vi "FUG-HCN.SetVoltage.vi"(0 "i ref in":refnum<vi>, 2 "Set Voltage":dbl format="%.5f", 4 "Time out":i32, 5 "error in (no error)":errorcluster) -> (14 "i ref out":refnum<vi>, 16 "timed out":bool, 19 "error out":errorcluster)   [LabVIEW 2014, in "FUG-HCN.lvlib"]
doc: "Sets the Voltage at the Device. but first one should increase the current to set the voltage else the Voltage might not be set"
uses:
  FUG-HCN.lvlib
  CS_Core/CSSystem/CoreLib/CoreLib.lvlib
  CS_Core/CSSystem/CoreDefs/CoreDefs.error_type.ctl
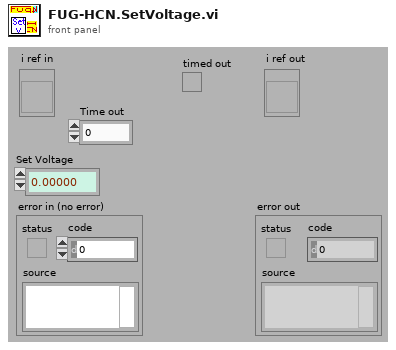
[diagram p1: front panel]
types:
  T1 = typedef "CoreDefs.error_type.ctl" = enum16{"no error", "can't load process", "can't unload process", "process does not exist", "can't install process", "can't remove process", "unknown function", "time out", "can't execute function", "duplicate queue name", "super not found", "caller queue invalid", "can't ping process", "unknown error", "VISA Error", "VISA timeout", "GPIB timeout", "GPIB error", "communication error", "data type mismatch", "can't read data from OPC server", "can't write data to OPC server", "OET error", "function not implemented", "process already exists", "invalid Shared Variable name", "error writing Shared Variable", "error reading Shared Variable", "invalid client name", "corrupt database", "unknown class", "call not authorized", "parameter out of range", "OET timeout: can't get data to modify", "invalid queue name", "requested operation incompatible with current state", "event undefined", "event disabled", "state undefined", "caller is not a friend", "EventBuilder: bad eventID", "EventBuilder: no DAQ devices", "a thread must not stop itself", "UNUSED ELEMENT4", "DiscArchiver: eventData incomplete", "DiscArchiver: eventData does not belong to run", "DiscArchiver: can't open file", "DiscArchiver: can't write to file", "DiscArchiver: available disc space low", "can't acquire semaphore", "error reading data from database", "notifier object is not existing", "can't register process", "can't unregister process", "illegal event type", "object disabled", "object already exists", "can't change state", "Instrument not found", "no connection to remote node", "invalid reference", "N/A", "UNUSED ELEMENT 1", "element not found", "illegal TCP/IP connection detected", "object does not exist", "invalid access ID", "unknown CS system", "invalid privilige", "unsupported data type", "unsupported server type", "IO server already exists", "Shared Variable already exists"}
  T2 = typedef "FUG-HCN.lvlib/FUG-HCN.i attribute.ctl" = cluster{"SetStatus":bool, "Set Voltage":dbl, "Nom Voltage":dbl, "VoltageID":i32, "CurrentID":i32}
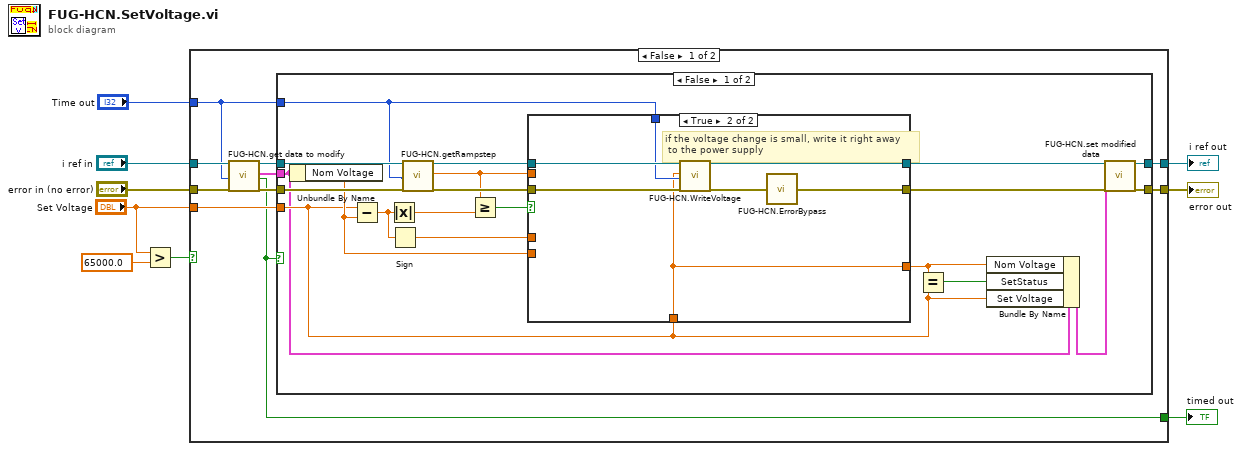
[diagram p0: block diagram]
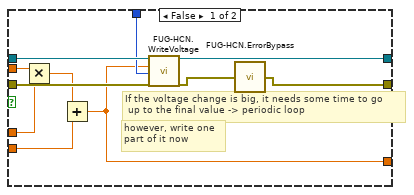
[diagram p2: hidden frame]
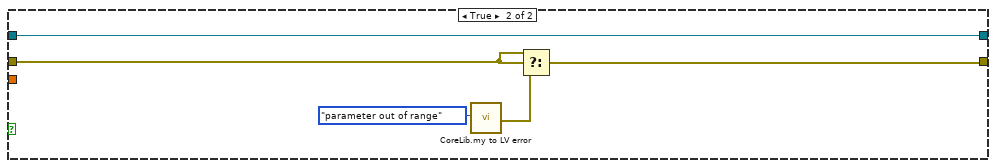
[diagram p4: hidden frame]
diagram:
  n1 = Greater?(x="Set Voltage", y=65000.0) -> (0:w2:bool)
  n2 = case shown="False" w2 {
    tunnel: [w19 w60] -> w9
    tunnel: "Set Voltage" -> [w18 _]
    tunnel: [w17 w64] -> w6
    tunnel: "i ref in" -> [w15 w64]
    tunnel: "error in (no error)" -> [w13 w62]
    tunnel: "Time out" -> [w14 _]
    tunnel: [w10 _] -> w1
    frame False {
      n3 = call "FUG-HCN.get data to modify.vi"("i ref in"=w15, "ms timeout (10000)"=w14, "error in (no error)"=w13) -> ("i ref out"=w16:refnum<vi>, "i attribute"=w11:T2, "timed out"=w10:bool, "error out"=w12:errorcluster)  [unwired: 13 in]
      n4 = case shown="False" w10 {
        tunnel: w11 -> [w22 _]
        tunnel: w12 -> [w33 w58]
        tunnel: [w35 w58] -> w19
        tunnel: w18 -> [w23 _]
        tunnel: w16 -> [w34 w59]
        tunnel: [w39 w59] -> w17
        tunnel: w14 -> [w24 _]
        frame False {
          n5 = Unbundle By Name(w22) -> ("Nom Voltage"=w25:dbl)
          n6 = Subtract(x=w23, y=w25) -> (x-y=w27:dbl)
          n7 = Absolute Value(x=w27) -> (abs(x)=w32:dbl)
          n8 = Sign(1:w27) -> (0:w26:dbl)
          n9 = call "FUG-HCN.getRampstep.vi"("i ref in"=w34, "ms timeout (100)"=w24, "error in (no error)"=w33) -> ("i ref out"=w29:refnum<vi>, "Ramp Step(V)"=w28:dbl, "error out"=w30:errorcluster)  [unwired: 13 in, 1 out]
          n10 = Greater Or Equal?(x=w28, y=w32) -> (x >= y?=w31:bool)
          n11 = case shown="True" w31 {
            tunnel: [w43 w54] -> w38
            tunnel: [w40 w51] -> w37
            tunnel: w30 -> [w49 w55]
            tunnel: w29 -> [w50 w57]
            tunnel: w24 -> [w48 w56]
            tunnel: w23 -> [_ w53]
            tunnel: w28 -> [w47 _]
            tunnel: w26 -> [w46 _]
            tunnel: w25 -> [w44 _]
            tunnel: [w42 w53] -> w21
            frame False {
              # "however, write one\npart of it now"
              # "If the voltage change is big, it needs some time to go\n up to the final value -> periodic loop"
              n12 = Multiply(x=w47, y=w46) -> (x*y=w45:dbl)
              n13 = Add(x=w45, y=w44) -> (x+y=w42:dbl)
              n14 = call "FUG-HCN.WriteVoltage.vi"("i ref in"=w50, "Set Voltage"=w42, "ms timeout (100)"=w48, "error in (no error)"=w49) -> ("i ref out"=w43:refnum<vi>, "error out"=w41:errorcluster)  [unwired: 13 in, 1 out]
              n15 = call "FUG-HCN.ErrorBypass.vi"("error in (no error)"=w41) -> ("error out"=w40:errorcluster)  [unwired: 14 in]
            }
            frame True {
              # "if the voltage change is small, write it right away\n to the power supply"
              n16 = call "FUG-HCN.WriteVoltage.vi"("i ref in"=w57, "Set Voltage"=w53, "ms timeout (100)"=w56, "error in (no error)"=w55) -> ("i ref out"=w54:refnum<vi>, "error out"=w52:errorcluster)  [unwired: 13 in, 1 out]
              n17 = call "FUG-HCN.ErrorBypass.vi"("error in (no error)"=w52) -> ("error out"=w51:errorcluster)  [unwired: 14 in]
            }
          }
          n18 = Equal?(x=w21, y=w23) -> (x = y?=w20:bool)
          n19 = Bundle By Name(cluster=w22, "Nom Voltage"=w21, "SetStatus"=w20, "Set Voltage"=w23) -> (w36:T2)
          n20 = call "FUG-HCN.set modified data.vi"("i ref in"=w38, "i attribute"=w36, "error in (no error)"=w37) -> ("i ref out"=w39:refnum<vi>, "error out"=w35:errorcluster)  [unwired: 15 in]
        }
        frame True {
        }
      }
    }
    frame True {
      n21 = call "CoreLib.my to LV error.vi"("ErrorTypes"=CoreDefs.error_type."parameter out of range") -> ("myErrorCluster"=w61:errorcluster)  [unwired: 17 in, 1 out]
      n22 = Select(t=w62, s=w62, f=w61) -> (s? t:f=w60:errorcluster)
    }
  }
  "error out" <- w9
  "i ref out" <- w6
  "timed out" <- w1
